vi "Handle Command.vi"(8 "error in":errorcluster, 10 "CMD in":refnum<class "Change Speaker Cycle Params.lvclass">, 11 "Object In":refnum<class>) -> (0 "error out":errorcluster, 1 "Command Successful?":bool, 2 "CMD out":refnum<class "Change Speaker Cycle Params.lvclass">, 3 "Object Out":refnum<class>)   [LabVIEW 2016, in "Change Speaker Cycle Params.lvclass"]
doc: "This VI will contain the code used to actually execute the request. If the request is successful, this will be indicated by the boolean output <b>Command Successful?</b>. The boolean output can then be used by the <b>Command Reply</b> which sends a reply if the reply queue is valid."
uses:
  Change Speaker Cycle Params.lvclass
  Main/PAS.lvclass
  G:/sw_repo/For Builds/Reusable/Instrument/Instrument.lvclass
  Instrument/Instrument.lvclass/Instrument.ctl
  Change Speaker Cycle Params.lvclass/Change Speaker Cycle Params.ctl
  Switch/Switch.lvclass/Switch.ctl
  Instrument/Read ExtCom.vi
  Switch/Write Cycle_.vi
  Main/Read Switch Ref.vi
  Switch/Write maxElapseTime.vi
  Main/Write Speaker Reference.vi
  Switch/Switch.lvclass
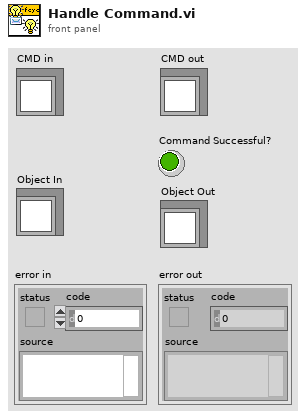
[diagram p1: front panel]
types:
  T1 = cluster{"tag":string, "section":string, "data":variant}
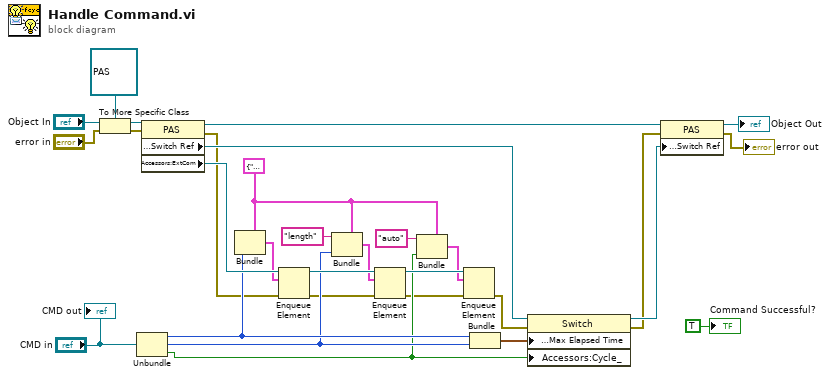
[diagram p0: block diagram]
diagram:
  w8 = T1 {"tag"="period", "section"="pas.spk", "data"=variant} ("element")
  n1 = To More Specific Class(target class=refnum<class "PAS.lvclass"> refnum ("PAS Library.lvlib:PAS"), reference="Object In", error in="error in") -> (specific class reference=w27:refnum<class "PAS.lvclass">, error out=w28:errorcluster)
  n2 = Unbundle("CMD in") -> (w15:u16, w11:u16, w6:bool)
  n3 = property class="PAS"(reference=w27, error in=w28) -> (reference out=w26:refnum<class "PAS.lvclass">, error out=w4:errorcluster, "Data Access:Switch Ref"=w25:refnum<class "Switch.lvclass">, "Accessors:ExtCom"=w16:refnum<queue>)
  n4 = Bundle(cluster=w8, "data"=w15) -> (w14:T1)  [unwired: 2 in]
  n5 = Enqueue Element(queue=w16, element=w14, error in (no error)=w4) -> (queue out=w13:refnum<queue>, error out=w3:errorcluster)  [unwired: 1 in, 1 out]
  n6 = Bundle(cluster=w8, "tag"="length", "data"=w11) -> (w10:T1)  [unwired: 1 in]
  n7 = Enqueue Element(queue=w13, element=w10, error in (no error)=w3) -> (queue out=w9:refnum<queue>, error out=w2:errorcluster)  [unwired: 1 in, 1 out]
  n8 = Bundle(cluster=w8, "tag"="auto", "data"=w6) -> (w5:T1)  [unwired: 1 in]
  n9 = Enqueue Element(queue=w9, element=w5, error in (no error)=w2) -> (error out=w1:errorcluster)  [unwired: 1 in, 2 out]
  n10 = Bundle("period"=w15, "length"=w11) -> (w22:cluster{"period":u16, "length":u16})  [unwired: 1 in]
  n11 = property class="Switch"(reference=w25, error in=w1, "Data Access:Max Elapsed Time"=w22, "Accessors:Cycle_"=w6) -> (reference out=w24:refnum<class "Switch.lvclass">, error out=w17:errorcluster)
  n12 = property class="PAS"(reference=w26, error in=w17, "Data Access:Switch Ref"=w24) -> (reference out=→"Object Out":refnum<class "PAS.lvclass">, error out=→"error out":errorcluster)
  "CMD out" <- "CMD in"
  "Command Successful?" <- TRUE ("Command Successful?")
